vi "Actor Core.vi"(8 "error in":errorcluster, 11 "Nested in":refnum<class "DAQ Controller.lvclass">) -> (0 "error out":errorcluster, 3 "Actor out":refnum<class "Actor.lvclass">)   [LabVIEW 2020, in "DAQ.lvlib" / "DAQ Controller.lvlib" / "DAQ Controller.lvclass"]
doc: "(<B>Filename</B>: Actor Framework.lvlib:Actor.lvclass:Actor Core.vi)\n\nReceives messages to the actor, reacts to them, and initiates any error handling that may shut the actor down.\n\nDescendant classes may override this VI to append parallel tasks for the actor to complete while it handles messages. Overrides use the Call Parent Method node."
uses:
  DAQ Controller.lvclass
  C:/Program Files/National Instruments/LabVIEW 2020/vi.lib/ActorFramework/Actor/Actor.lvclass
  <vilib>/ActorFramework/Actor/Actor.lvclass
  DAQ Controller.lvclass/DAQ Controller.ctl
  <vilib>/ActorFramework/Actor/Actor.lvclass/Actor.ctl
  <vilib>/ActorFramework/Message Enqueuer/Message Enqueuer.lvclass/Message Enqueuer.ctl
  Real Hardware/DAQ_QPT_Throlab/DAQ_QPT_Throlab Messages/Start TIRF Locked Msg/Start TIRF Locked Msg.lvclass/Start TIRF Locked Msg.ctl
  <vilib>/ActorFramework/Message Enqueuer/Init from Existing Queue.vi
  <vilib>/ActorFramework/Message Enqueuer/Enqueue.vi
  Real Hardware/DAQ_QPT_Throlab/DAQ_QPT_Throlab Messages/Start TIRF Locked Msg/Start TIRF Locked Msg.lvclass
  C:/Program Files/National Instruments/LabVIEW 2020/vi.lib/ActorFramework/Message/Message.lvclass
  <vilib>/ActorFramework/Stop Msg/Stop Msg.lvclass
  <vilib>/ActorFramework/Message Priority Queue/Priority Enqueue.vi
  <vilib>/ActorFramework/Message Enqueuer/Message Enqueuer.lvclass
panel:
  in  "Tirf_Locked":bool
  out "QPD Y":dbl(graph)
  out "QPD X":dbl(graph)
  out "Sum":dbl
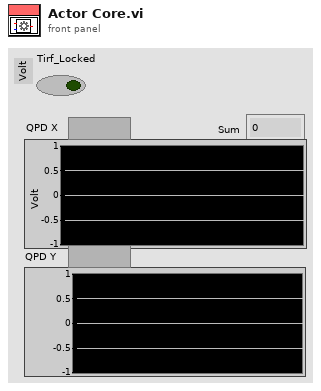
[diagram p1: front panel]
types:
  T1 = cluster{"Stop":refnum<user-event>, "QPD X":refnum<user-event>, "QPD Y":refnum<user-event>, "Sum":refnum<user-event>}
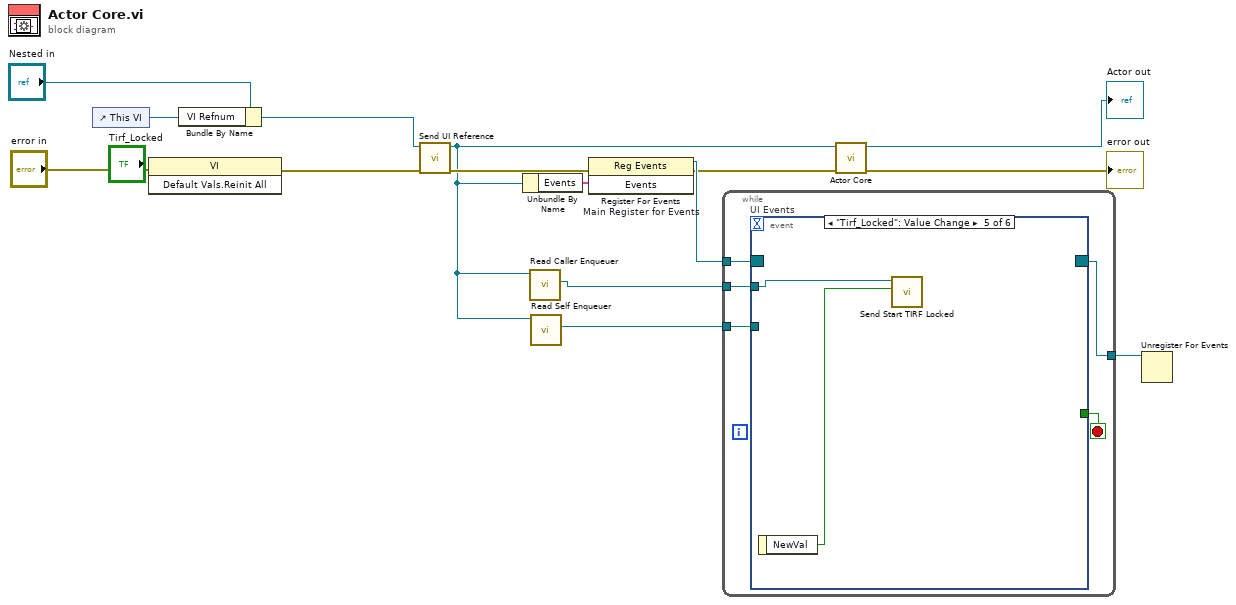
[diagram p0: block diagram]
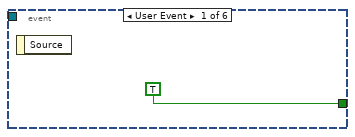
[diagram p2: hidden frame]
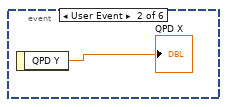
[diagram p3: hidden frame]
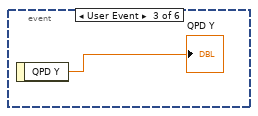
[diagram p4: hidden frame]
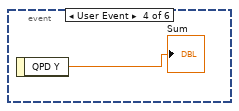
[diagram p5: hidden frame]
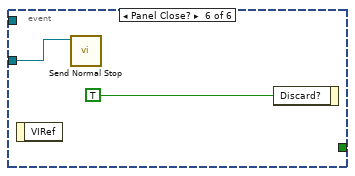
[diagram p6: hidden frame]
diagram:
  n1 = control-ref of="This VI"() -> (w5:refnum<vi>)
  n2 = invoke class="VI" method="Default Vals.Reinit All"(error in="error in") -> (error out=w7:errorcluster)  [unwired: 2 in, 2 out]
  n3 = Bundle By Name(cluster="Nested in", "VI Refnum"=w5) -> (w3:refnum<class "DAQ Controller.lvclass">)
  n4 = call-dynamic "Send UI Reference.vi"("error in (no error)"=w7, "DAQ Controller in"=w3) -> ("error out"=w4:errorcluster, "DAQ Controller out"=w2:refnum<class "DAQ Controller.lvclass">)  [unwired: 8 in]
  n5 = Unbundle By Name(w2) -> ("Events"=w12:T1)
  n6 = call <vilib>:"Read Caller Enqueuer.vi"("Actor"=w2) -> ("Caller Enqueuer"=w1:refnum<class "Message Enqueuer.lvclass">)  [unwired: 10 in]
  n7 = call <vilib>:"Read Self Enqueuer.vi"("Actor"=w2) -> ("Self Enqueuer"=w9:refnum<class "Message Enqueuer.lvclass">)  [unwired: 10 in]
  n8 = register-events "Main Register for Events"(error in=w4, w12) -> (reference out=w13:refnum<event-registration>, error out=w8:errorcluster)  [unwired: 1 in]
  n9 = while {
    tunnel: w13 -> [w20]
    tunnel: [w18] -> w11
    tunnel: w9 -> [w17]
    tunnel: w1 -> [w16]
    stop <- w19 stop-if-true
    n10 = event "UI Events" shown="[4] \"Tirf_Locked\": Value Change" {
      selector: w20 -> [_ _ _ _ _ _]
      dyn-events: [_ _ _ _ _ _] -> w18
      timeout: _ -> [_ _ _ _ _ _]
      tunnel: [TRUE _ _ _ _ _] -> w19
      tunnel: w17 -> [_ _ _ _ _ w27]
      tunnel: w16 -> [_ _ _ _ w26 _]
      event User Event {
        n11 = event-data() -> ()  [unwired: 1 in, 1 out]
      }
      event User Event {
        n12 = event-data() -> ("QPD Y"=→"QPD X":dbl)  [unwired: 1 in]
      }
      event User Event {
        n13 = event-data() -> ("QPD Y"=→"QPD Y":dbl)  [unwired: 1 in]
      }
      event User Event {
        n14 = event-data() -> ("QPD Y"=→"Sum":dbl)  [unwired: 1 in]
      }
      event "Tirf_Locked": Value Change {
        n15 = event-data() -> ("NewVal"=w25:bool)  [unwired: 1 in]
        n16 = call "Send Start TIRF Locked.vi"("TIRF Locked?"=w25, "Message Enqueuer"=w26) -> ()  [unwired: 8 in, 2 out]
      }
      event Panel Close? {
        n17 = event-data() -> ()  [unwired: 1 in, 1 out]
        n18 = call <vilib>:"Send Normal Stop.vi"("Message Enqueuer"=w27) -> ()  [unwired: 10 in, 1 out]
        n19 = event-data("Discard?"=TRUE) -> ()  [unwired: 1 in, 1 out]
      }
    }
  }
  n20 = call-parent "Actor Core.vi"("error in"=w8, "Actor in"=w2) -> ("error out"=→"error out":errorcluster, "Actor out"=→"Actor out":refnum<class "Actor.lvclass">)  [unwired: 8 in]
  n21 = Unregister For Events(event registration refnum=w11) -> ()  [unwired: 1 in, 1 out]
